vi "Untitled 1.vi"() -> ()   [LabVIEW 2020]
uses:
  <vilib>/Instr/_visa.llb/VISA Configure Serial Port (Instr).vi
panel:
  in  "stop":bool
  in  "Strb":bool
  in  "Bcn":bool
  in  "Tax":bool
  in  "Land":bool
  in  "Nav":bool
  in  "VISA resource name":refnum<visa-resource-name>
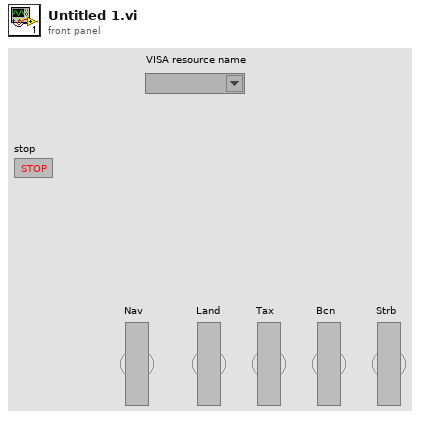
[diagram p1: front panel]
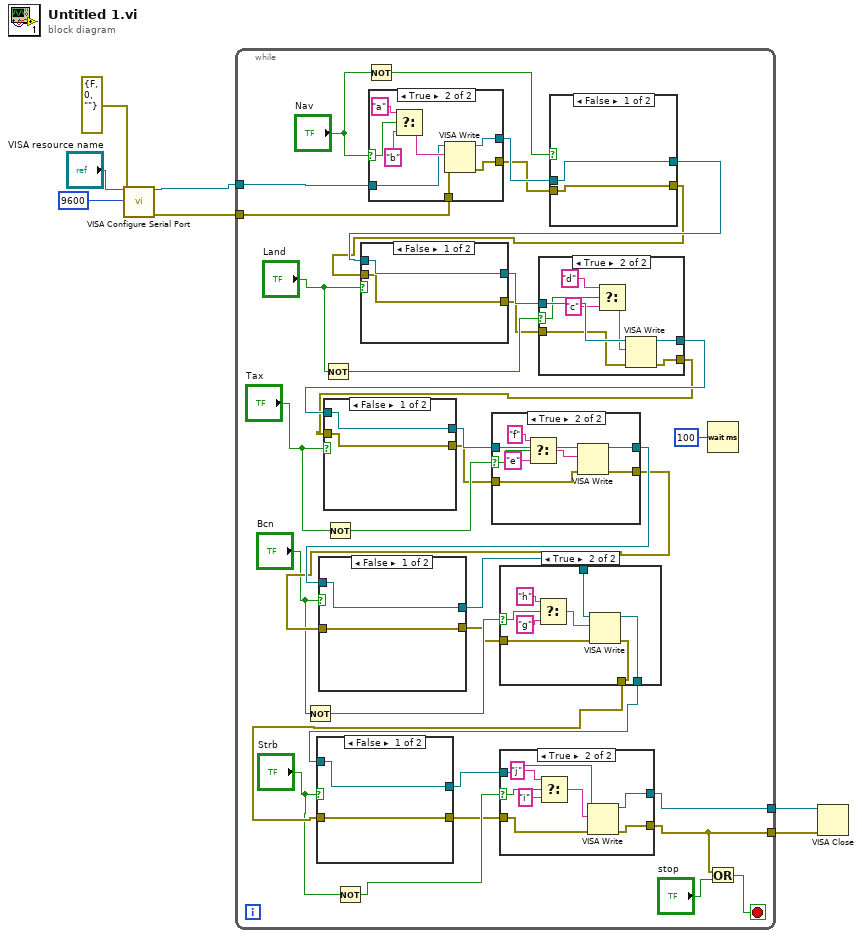
[diagram p0: block diagram]
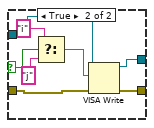
[diagram p3: hidden frame]
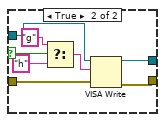
[diagram p5: hidden frame]
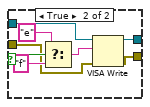
[diagram p7: hidden frame]
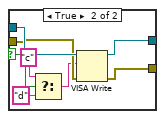
[diagram p9: hidden frame]
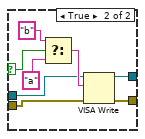
[diagram p10: hidden frame]
diagram:
  n1 = call-poly "VISA Configure Serial Port"("VISA resource name"="VISA resource name", "baud rate (9600)"=u32 9600, "error in (no error)"=errorcluster {"status"=FALSE, "code"=0, "source"=""}) -> ("VISA resource name out"=w5:refnum<visa-resource-name>, "error out"=w4:errorcluster)  [unwired: 11 in]
  n2 = while {
    tunnel: w5 -> [w42]
    tunnel: w4 -> [w41]
    tunnel: [w12] -> w3
    tunnel: [w10] -> w2
    stop <- w9 stop-if-true
    n3 = Not(x="Bcn") -> (.not. x?=w21:bool)
    n4 = Not(x="Land") -> (.not. x?=w33:bool)
    n5 = Not(x="Tax") -> (.not. x?=w27:bool)
    n6 = Not(x="Strb") -> (.not. x?=w15:bool)
    n7 = Not(x="Nav") -> (.not. x?=w39:bool)
    n8 = case shown="True" "Nav" {
      selector: "Nav" -> [_ w139]
      tunnel: w42 -> [w134 w138]
      tunnel: w41 -> [w133 w137]
      tunnel: [w134 w136] -> w38
      tunnel: [w133 w135] -> w37
      frame False {
      }
      frame True {
        n9 = Select(t="a", s=w139, f="b") -> (s? t:f=w142:string)
        n10 = VISA Write(VISA resource name=w138, write buffer=w142, error in (no error)=w137) -> (VISA resource name out=w136:refnum<visa-resource-name>, error out=w135:errorcluster)  [unwired: 1 out]
      }
    }
    n11 = case shown="False" w39 {
      selector: w39 -> [_ w132]
      tunnel: w38 -> [w124 w128]
      tunnel: w37 -> [w123 w127]
      tunnel: [w124 w126] -> w36
      tunnel: [w123 w125] -> w35
      frame False {
      }
      frame True {
        n12 = Select(t="b", s=w132, f="a") -> (s? t:f=w129:string)
        n13 = VISA Write(VISA resource name=w128, write buffer=w129, error in (no error)=w127) -> (VISA resource name out=w126:refnum<visa-resource-name>, error out=w125:errorcluster)  [unwired: 1 out]
      }
    }
    n14 = case shown="False" "Land" {
      selector: "Land" -> [_ w120]
      tunnel: w36 -> [w114 w122]
      tunnel: w35 -> [w113 w121]
      tunnel: [w114 w116] -> w32
      tunnel: [w113 w115] -> w31
      frame False {
      }
      frame True {
        n15 = Select(t="c", s=w120, f="d") -> (s? t:f=w117:string)
        n16 = VISA Write(VISA resource name=w122, write buffer=w117, error in (no error)=w121) -> (VISA resource name out=w116:refnum<visa-resource-name>, error out=w115:errorcluster)  [unwired: 1 out]
      }
    }
    n17 = case shown="True" w33 {
      selector: w33 -> [_ w110]
      tunnel: w32 -> [w104 w112]
      tunnel: w31 -> [w103 w111]
      tunnel: [w104 w106] -> w30
      tunnel: [w103 w105] -> w29
      frame False {
      }
      frame True {
        n18 = Select(t="d", s=w110, f="c") -> (s? t:f=w107:string)
        n19 = VISA Write(VISA resource name=w112, write buffer=w107, error in (no error)=w111) -> (VISA resource name out=w106:refnum<visa-resource-name>, error out=w105:errorcluster)  [unwired: 1 out]
      }
    }
    n20 = case shown="False" "Tax" {
      selector: "Tax" -> [_ w102]
      tunnel: w30 -> [w94 w98]
      tunnel: w29 -> [w93 w97]
      tunnel: [w94 w96] -> w26
      tunnel: [w93 w95] -> w25
      frame False {
      }
      frame True {
        n21 = Select(t="e", s=w102, f="f") -> (s? t:f=w99:string)
        n22 = VISA Write(VISA resource name=w98, write buffer=w99, error in (no error)=w97) -> (VISA resource name out=w96:refnum<visa-resource-name>, error out=w95:errorcluster)  [unwired: 1 out]
      }
    }
    n23 = case shown="True" w27 {
      selector: w27 -> [_ w90]
      tunnel: w26 -> [w84 w92]
      tunnel: w25 -> [w83 w91]
      tunnel: [w84 w86] -> w24
      tunnel: [w83 w85] -> w23
      frame False {
      }
      frame True {
        n24 = Select(t="f", s=w90, f="e") -> (s? t:f=w87:string)
        n25 = VISA Write(VISA resource name=w92, write buffer=w87, error in (no error)=w91) -> (VISA resource name out=w86:refnum<visa-resource-name>, error out=w85:errorcluster)  [unwired: 1 out]
      }
    }
    n26 = case shown="False" "Bcn" {
      selector: "Bcn" -> [_ w82]
      tunnel: w24 -> [w74 w78]
      tunnel: w23 -> [w73 w77]
      tunnel: [w74 w76] -> w20
      tunnel: [w73 w75] -> w19
      frame False {
      }
      frame True {
        n27 = Select(t="g", s=w82, f="h") -> (s? t:f=w79:string)
        n28 = VISA Write(VISA resource name=w78, write buffer=w79, error in (no error)=w77) -> (VISA resource name out=w76:refnum<visa-resource-name>, error out=w75:errorcluster)  [unwired: 1 out]
      }
    }
    n29 = case shown="True" w21 {
      selector: w21 -> [_ w72]
      tunnel: w20 -> [w64 w68]
      tunnel: w19 -> [w63 w67]
      tunnel: [w64 w66] -> w18
      tunnel: [w63 w65] -> w17
      frame False {
      }
      frame True {
        n30 = Select(t="h", s=w72, f="g") -> (s? t:f=w69:string)
        n31 = VISA Write(VISA resource name=w68, write buffer=w69, error in (no error)=w67) -> (VISA resource name out=w66:refnum<visa-resource-name>, error out=w65:errorcluster)  [unwired: 1 out]
      }
    }
    n32 = case shown="False" "Strb" {
      selector: "Strb" -> [_ w62]
      tunnel: w18 -> [w54 w58]
      tunnel: w17 -> [w53 w57]
      tunnel: [w54 w56] -> w14
      tunnel: [w53 w55] -> w13
      frame False {
      }
      frame True {
        n33 = Select(t="i", s=w62, f="j") -> (s? t:f=w59:string)
        n34 = VISA Write(VISA resource name=w58, write buffer=w59, error in (no error)=w57) -> (VISA resource name out=w56:refnum<visa-resource-name>, error out=w55:errorcluster)  [unwired: 1 out]
      }
    }
    n35 = case shown="True" w15 {
      selector: w15 -> [_ w52]
      tunnel: w14 -> [w44 w48]
      tunnel: w13 -> [w43 w47]
      tunnel: [w44 w46] -> w12
      tunnel: [w43 w45] -> w10
      frame False {
      }
      frame True {
        n36 = Select(t="j", s=w52, f="i") -> (s? t:f=w49:string)
        n37 = VISA Write(VISA resource name=w48, write buffer=w49, error in (no error)=w47) -> (VISA resource name out=w46:refnum<visa-resource-name>, error out=w45:errorcluster)  [unwired: 1 out]
      }
    }
    n38 = Wait (ms)(milliseconds to wait=u32 100) -> ()  [unwired: 1 out]
    n39 = Or(x=w10, y="stop") -> (x .or. y?=w9:bool)
  }
  n40 = VISA Close(VISA resource name=w3, error in (no error)=w2) -> ()  [unwired: 1 out]
